vi "Open API Reference.vi"(8 "error in (no error)":errorcluster) -> (0 "error out":errorcluster, 3 "Execution API out":refnum<class "Execution API.lvclass">)   [LabVIEW 2020, in "Execution API.lvclass"]
uses:
  Execution API.lvclass
  C:/Users/anton/Documents/GitHub/LUnit/source/Application Framework/Process Classes/Process/Process.lvclass
  Application Framework/Process Classes/Process/Process.lvclass
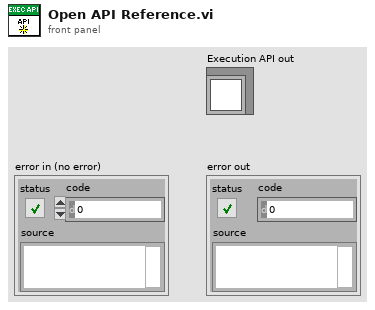
[diagram p1: front panel]
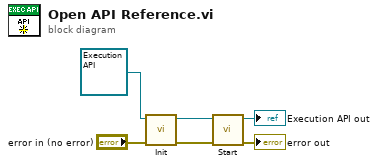
[diagram p0: block diagram]
diagram:
  n1 = call-dynamic "Init.vi"("error in (no error)"="error in (no error)", "Execution API In"=refnum<class "Execution API.lvclass"> refnum ("LUnit API.lvclass")) -> ("error out"=w2:errorcluster, "Execution API Out"=w3:refnum<class "Execution API.lvclass">)  [unwired: 8 in]
  n2 = call "Start.vi"("error in (no error)"=w2, "Process In"=w3) -> ("error out"=→"error out":errorcluster, "Process Out"=→"Execution API out":refnum<class "Execution API.lvclass">)  [unwired: 8 in]
